vi "Modem Status Write Data.vi"(8 "error in (no error)":errorcluster, 10 "CMD ID":u8, 11 "VISA Refnum in":refnum<visa-resource-name>) -> (0 "error out":errorcluster, 3 "VISA Refnum out":refnum<visa-resource-name>)   [LabVIEW 2011]
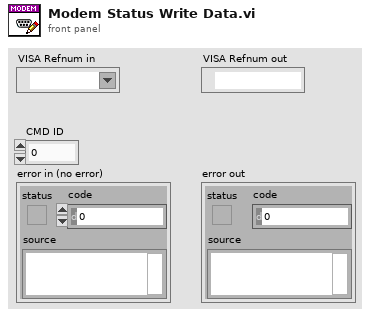
[diagram p1: front panel]
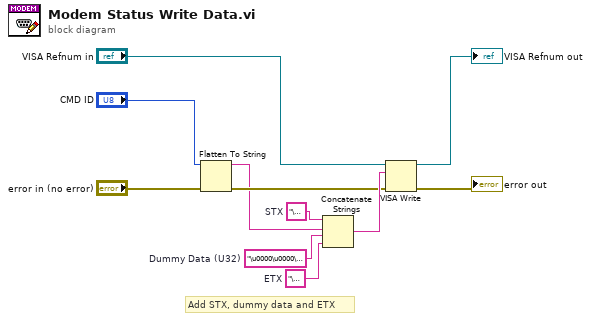
[diagram p0: block diagram]
diagram:
  w2 = "\u0000\u0000\u0000\u0000"  # Dummy Data (U32)
  w7 = "\u0003"  # ETX
  w6 = "\u0002"  # STX
  # "Add STX, dummy data and ETX"
  n1 = Flatten To String(anything="CMD ID", error in (no error)="error in (no error)") -> (data string=w1:string, error out=w3:errorcluster)  [unwired: 2 in, 1 out]
  n2 = Concatenate Strings(w6, w1, w2, w7) -> (w8:string)
  n3 = VISA Write(VISA resource name="VISA Refnum in", write buffer=w8, error in (no error)=w3) -> (VISA resource name out=→"VISA Refnum out":refnum<visa-resource-name>, error out=→"error out":errorcluster)  [unwired: 1 out]
